vi "ReadConfigTemp.vi"(2 "Error In":errorcluster, 3 "Configs":string) -> (0 "Error Out":errorcluster, 1 "ConfigTemps":T1[](array[typedef]))   [LabVIEW 2012]
uses:
  TempConfig.ctl
  <vilib>/LVH/i3 JSON/i3-json.lvlib
panel:
  in  "tempTable":cluster{"ConfigTemps":T1[]}
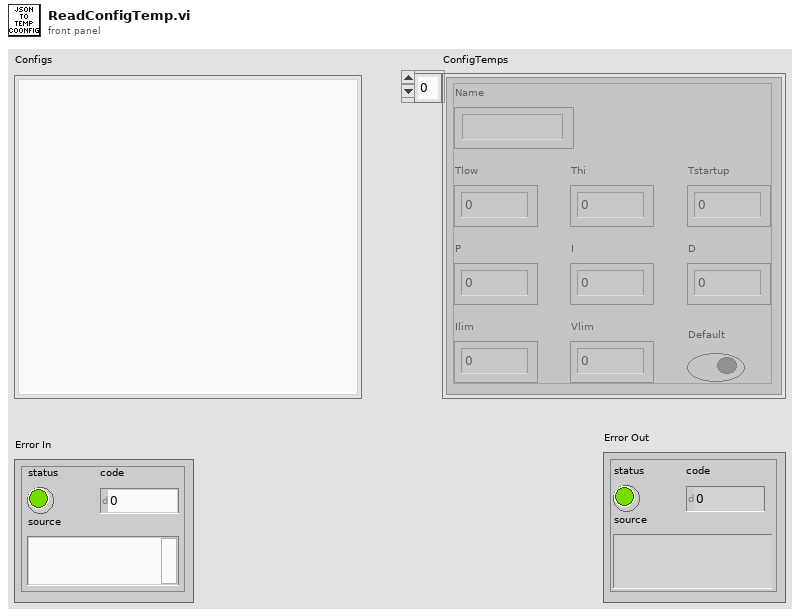
[diagram p1: front panel]
types:
  T1 = typedef "TempConfig.ctl" = cluster{"Name":string, "Thi":dbl, "Tlow":dbl, "Tstartup":dbl, "P":dbl, "I":dbl, "D":dbl, "Ilim":dbl, "Vlim":dbl, "Default":bool}
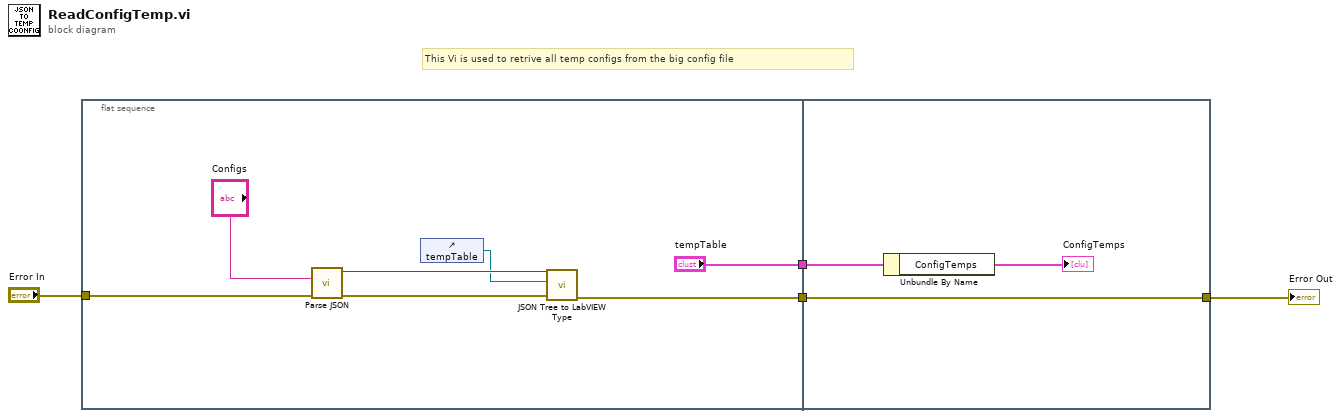
[diagram p0: block diagram]
diagram:
  # "This Vi is used to retrive all temp configs from the big config file"
  n1 = flat-sequence {
    tunnel: "Error In" -> [w7]
    tunnel: [w6] -> w2
    tunnel: ["tempTable"] -> w1
    tunnel: [w13] -> w3
    tunnel: w2 -> [w13]
    tunnel: w1 -> [w12]
    frame #0 {
      n2 = call <vilib>:"Parse JSON.vi"("error in (no error)"=w7, "JSON String"="Configs") -> ("error out"=w10:errorcluster, "JSON Tree"=w11:variant)  [unwired: 6 in, 2 out]
      n3 = control-ref of="tempTable"() -> (w8:refnum<vi>)
      n4 = call <vilib>:"JSON Tree to LabVIEW Type.vi"("error in (no error)"=w10, "Ctl Refnum"=w8, "JSON Tree In"=w11) -> ("error out"=w6:errorcluster)  [unwired: 7 in, 1 out]
    }
    frame #1 {
      n5 = Unbundle By Name(w12) -> ("ConfigTemps"=→"ConfigTemps":T1[])
    }
  }
  "Error Out" <- w3
